vi "Dispose.vi"(8 "error in (no error)":errorcluster, 11 "EnchantedRoom":refnum<class "EnchantedRoom.lvclass">) -> (0 "error out":errorcluster)   [LabVIEW 2020, in "EnchantedRoom.lvclass"]
uses:
  EnchantedRoom.lvclass
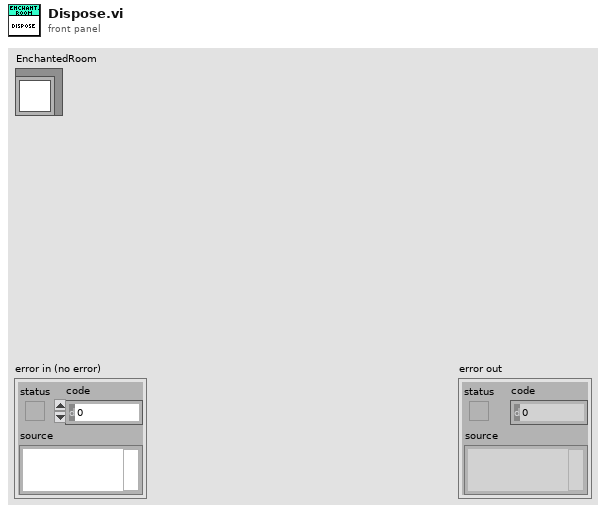
[diagram p1: front panel]
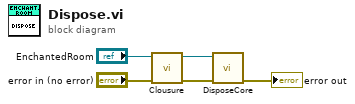
[diagram p0: block diagram]
diagram:
  n1 = call-dynamic "Clousure.vi"("error in (no error)"="error in (no error)", "EnchantedRoom"="EnchantedRoom") -> ("error out"=w5:errorcluster, "EnchantedRoom"=w4:refnum<class "EnchantedRoom.lvclass">)  [unwired: 8 in]
  n2 = call-dynamic "DisposeCore.vi"("error in (no error)"=w5, "EnchantedRoom"=w4) -> ("error out"=→"error out":errorcluster)  [unwired: 8 in, 1 out]
